vi "Waveform Edit.vi"(6 "Change in Time":i32, 9 "In Use Cluster":T1, 10 "New Data":dbl[][](array[numeric]), 11 "Old Data":dbl[][](array[numeric])) -> (1 "Overview Chart Data":waveform(dbl)[](array[waveform]), 2 "Output Waveform Cluster":T2, 3 "Output Decimated Data":dbl[][](array[numeric]))   [LabVIEW 2014]
panel:
  # "Waveform Edit VI"
  # "Inputs"
  # "Outputs"
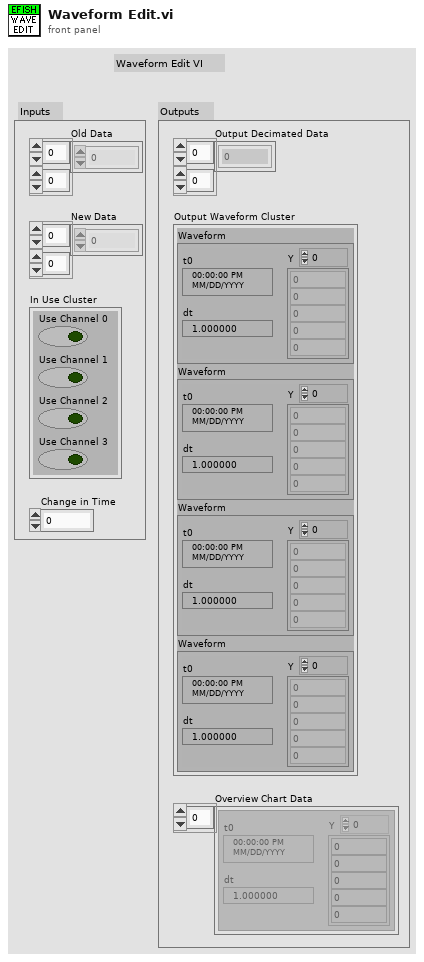
[diagram p1: front panel]
types:
  T1 = cluster{"Use Channel 0":bool, "Use Channel 1":bool, "Use Channel 2":bool, "Use Channel 3":bool}
  T2 = cluster{"Waveform":waveform(dbl), "Waveform":waveform(dbl), "Waveform":waveform(dbl), "Waveform":waveform(dbl)}
  T3 = cluster{"New Data":dbl[], "Old Data":dbl[], i32, dbl, "Use Channel 1":bool}
  T4 = cluster{"New Data":dbl[], "Old Data":dbl[], i32, dbl, "Use Channel 2":bool}
  T5 = cluster{"New Data":dbl[], "Old Data":dbl[], i32, dbl, "Use Channel 3":bool}
  T6 = cluster{"New Data":dbl[], "Old Data":dbl[], i32, dbl, "Use Channel 0":bool}
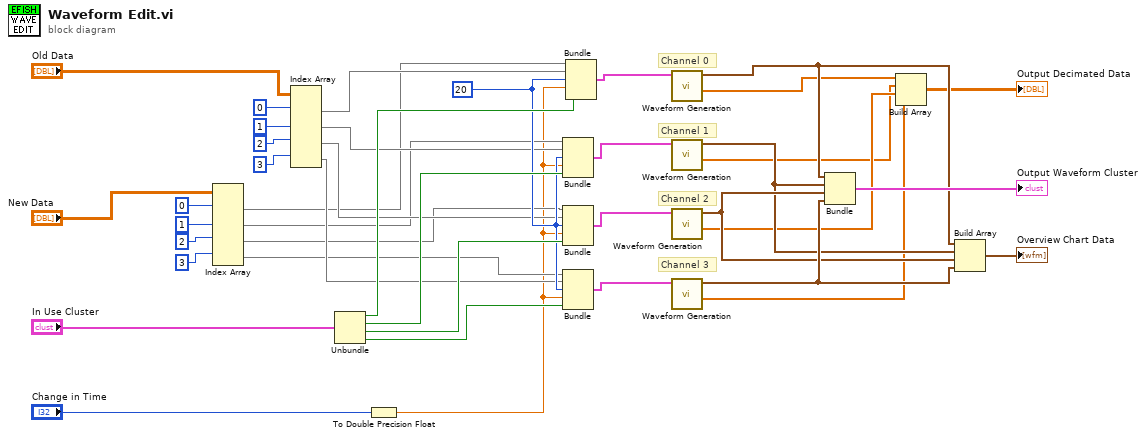
[diagram p0: block diagram]
diagram:
  w21 = 20
  # "Channel 3"
  # "Channel 2"
  # "Channel 1"
  # "Channel 0"
  n1 = Index Array(array="New Data", index (row) #1=0 ("index (row)"), index (row) #2=1 ("index (row)"), index (row) #3=2 ("index (row)"), index (row) #4=3 ("index (row)")) -> (element #1=w5:dbl[], element #2=w4:dbl[], element #3=w3:dbl[], element #4=w2:dbl[])  [unwired: 4 in]
  n2 = Index Array(array="Old Data", index (row) #1=0 ("index (row)"), index (row) #2=1 ("index (row)"), index (row) #3=2 ("index (row)"), index (row) #4=3 ("index (row)")) -> (element #1=w17:dbl[], element #2=w13:dbl[], element #3=w12:dbl[], element #4=w11:dbl[])  [unwired: 4 in]
  n3 = Unbundle("In Use Cluster") -> ("Use Channel 0"=w23:bool, "Use Channel 1"=w24:bool, "Use Channel 2"=w25:bool, "Use Channel 3"=w26:bool)
  n4 = To Double Precision Float(number="Change in Time") -> (double precision float=w1:dbl)
  n5 = Bundle("New Data"=w4, "Old Data"=w13, w21, w1, "Use Channel 1"=w24) -> (w29:T3)  [unwired: 1 in]
  n6 = Bundle("New Data"=w3, "Old Data"=w12, w21, w1, "Use Channel 2"=w25) -> (w28:T4)  [unwired: 1 in]
  n7 = Bundle("New Data"=w2, "Old Data"=w11, w21, w1, "Use Channel 3"=w26) -> (w27:T5)  [unwired: 1 in]
  n8 = Bundle("New Data"=w5, "Old Data"=w17, w21, w1, "Use Channel 0"=w23) -> (w30:T6)  [unwired: 1 in]
  n9 = call "Waveform Generation.vi"("Cluster"=w30) -> ("Output Y Values"=w31:dbl[], "Waveform"=w37:waveform(dbl))  [unwired: 9 in]
  n10 = call "Waveform Generation.vi"("Cluster"=w29) -> ("Output Y Values"=w32:dbl[], "Waveform"=w38:waveform(dbl))  [unwired: 9 in]
  n11 = call "Waveform Generation.vi"("Cluster"=w28) -> ("Output Y Values"=w33:dbl[], "Waveform"=w39:waveform(dbl))  [unwired: 9 in]
  n12 = call "Waveform Generation.vi"("Cluster"=w27) -> ("Output Y Values"=w34:dbl[], "Waveform"=w40:waveform(dbl))  [unwired: 9 in]
  n13 = Bundle("Waveform"=w37, "Waveform"=w38, "Waveform"=w39, "Waveform"=w40) -> (→"Output Waveform Cluster":T2)  [unwired: 1 in]
  n14 = Build Array(w31, w32, w33, w34) -> (→"Output Decimated Data":dbl[][])
  n15 = Build Array(w37, w38, w39, w40) -> (→"Overview Chart Data":waveform(dbl)[])
